vi "GetGamePiece.vi"() -> (0 "tx":dbl, 1 "ty":dbl, 2 "piece?":string, 3 "Vision Target Valid [t-?]":bool, 4 "confidence":dbl, 6 "Vision Timestamp (ms)":u32)   [LabVIEW 2020]
doc: "Reads the raw data from the LimeLight camera assigned to detecting AprilTags. Performs some minor transformations, conducts intial validity checks, and estimates the vision data timestamp."
uses:
  2d64956e-cf35-4d84-838e-e30eff74bf58.vi
  <vilib>/Rock Robotics/Network Tables/NT Read Number.vi
  GlobalDriverStationData.vi
  <vilib>/Rock Robotics/Network Tables/NT Read Numeric Array.vi
  <vilib>/Rock Robotics/Network Tables/NT Read String.vi
  GlobalPoseAndTargeting.vi
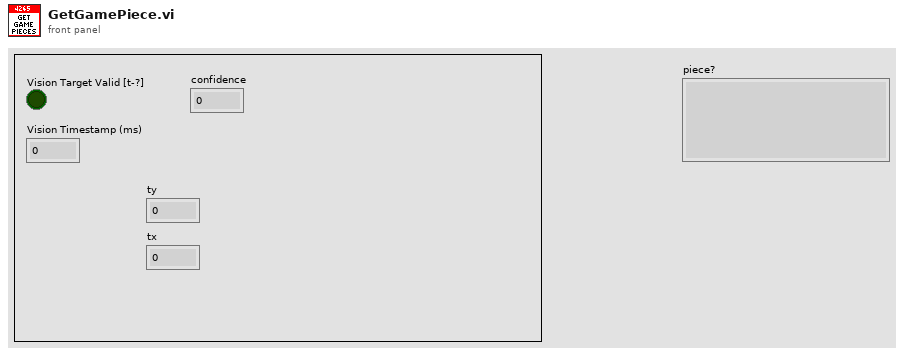
[diagram p1: front panel]
types:
  T1 = enum16{"Boot Up", "Camera Override", "AprilTags", "Gamepiece Tracking"}
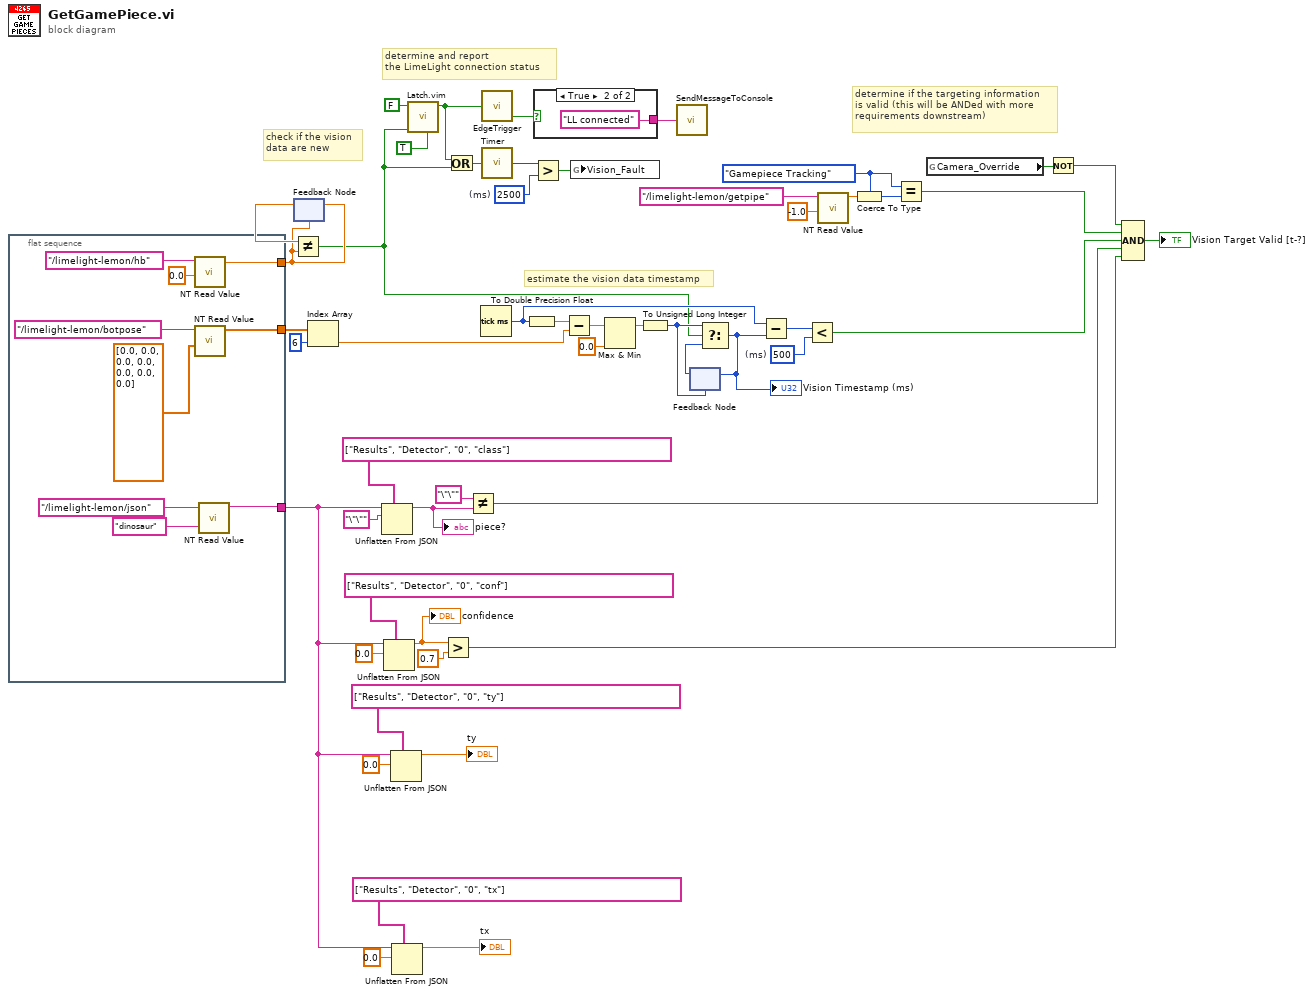
[diagram p0: block diagram]
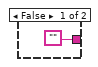
[diagram p2: hidden frame]
diagram:
  w24 = T1."Gamepiece Tracking"
  w35 = u32 2500  # (ms)
  w28 = u32 500  # (ms)
  # "determine and report\nthe LimeLight connection status"
  # "determine if the targeting information\nis valid (this will be ANDed with more\nrequirements downstream)"
  # "estimate the vision data timestamp"
  # "check if the vision\ndata are new"
  n1 = flat-sequence {
    tunnel: [w59] -> w26
    tunnel: [w56] -> w21
    tunnel: [w54] -> w1
    frame #0 {
      n2 = call-poly <vilib>:"NT Read Value.vi"("default value"=0.0 ("Default Value"), "name"="/limelight-lemon/hb" ("Name")) -> ("value"=w59:dbl)  [unwired: 7 in, 2 out]
      n3 = call-poly <vilib>:"NT Read Value.vi"("default value"=dbl[] [0.0, 0.0, 0.0, 0.0, 0.0, 0.0, 0.0], "name"="/limelight-lemon/botpose" ("Name")) -> ("value"=w56:dbl[])  [unwired: 7 in, 2 out]
      n4 = call-poly <vilib>:"NT Read Value.vi"("default value"="dinosaur", "name"="/limelight-lemon/json" ("Name")) -> ("value"=w54:string)  [unwired: 7 in, 2 out]
    }
  }
  n5 = feedback-in #1(w26) -> ()
  n6 = feedback #1(w26) -> (w37:dbl)
  n7 = Not Equal?(x=w37, y=w26) -> (x != y?=w25:bool)
  n8 = Index Array(array=w21, index=6) -> (element=w20:dbl)
  n9 = Unflatten From JSON(path=string[] ["Results", "Detector", "0", "class"], JSON string=w1, type and defaults="\"\"") -> (value=w2:string)  [unwired: 4 in, 1 out]
  "piece?" <- w2
  n10 = Unflatten From JSON(path=string[] ["Results", "Detector", "0", "conf"], JSON string=w1, type and defaults=0.0) -> (value=w10:dbl)  [unwired: 4 in, 1 out]
  "confidence" <- w10
  n11 = Unflatten From JSON(path=string[] ["Results", "Detector", "0", "ty"], JSON string=w1, type and defaults=0.0) -> (value=→"ty":dbl)  [unwired: 4 in, 1 out]
  n12 = Unflatten From JSON(path=string[] ["Results", "Detector", "0", "tx"], JSON string=w1, type and defaults=0.0) -> (value=→"tx":dbl)  [unwired: 4 in, 1 out]
  n13 = call "Latch.vim"("Default Value"=TRUE, "Latch Signal"=w25, "Latch Value"=FALSE) -> ("Latched"=w31:bool)  [unwired: 8 in]
  n14 = Greater?(x=w10, y=0.7 ("x")) -> (0:w12:bool)
  n15 = Or(x=w31, y=w25) -> (x .or. y?=w34:bool)
  n16 = Not Equal?(x="\"\"", y=w2) -> (x != y?=w3:bool)
  n17 = Tick Count (ms)() -> (millisecond timer value=w41:u32)
  n18 = call "EdgeTrigger.vi"("Input Signal"=w31) -> ("Falling Edge Trigger"=w29:bool)  [unwired: 2 out]
  n19 = call "Timer.vi"("Reset Timer"=w34) -> ("Time (ms)"=w36:u32)
  n20 = To Double Precision Float(number=w41) -> (double precision float=w46:dbl)
  n21 = Greater?(x=w36, y=w35) -> (0:w27:bool)
  n22 = case shown="True" w29 {
    tunnel: ["" "LL connected" ("Message")] -> w30
    frame False {
    }
    frame True {
    }
  }
  n23 = Subtract(x=w46, y=w20) -> (x-y=w45:dbl)
  n24 = global write "GlobalPoseAndTargeting.vi" "Vision_Fault"(w27) -> ()
  n25 = Max & Min(x=w45, y=0.0) -> (max(x,y)=w43:dbl)  [unwired: 1 out]
  n26 = To Unsigned Long Integer(number=w43) -> (unsigned 32bit integer=w42:u32)
  n27 = call "SendMessageToConsole.vi"("Message String"=w30) -> ()  [unwired: 1 in]
  n28 = feedback #2(w42) -> (w47:u32)
  n29 = Select(t=w42, s=w25, f=w47) -> (s? t:f=w18:u32)
  "Vision Timestamp (ms)" <- w18
  n30 = feedback-in #2(w18) -> ()
  n31 = Subtract(x=w41, y=w18) -> (x-y=w40:u32)
  n32 = Less?(x=w40, y=w28) -> (x < y?=w23:bool)
  n33 = call-poly <vilib>:"NT Read Value.vi"("default value"=-1.0 ("Default Value"), "name"="/limelight-lemon/getpipe" ("Name")) -> ("value"=w50:dbl)  [unwired: 7 in, 2 out]
  n34 = Coerce To Type(0:w50, 1:w24) -> (2:w49:T1)
  n35 = Equal?(x=w24, y=w49) -> (x = y?=w48:bool)
  n36 = global read "GlobalDriverStationData.vi" "Camera_Override"() -> (w39:bool)
  n37 = Not(x=w39) -> (.not. x?=w38:bool)
  n38 = Compound Arithmetic op=AND(w38, w48, w23, w3, w12) -> (→"Vision Target Valid [t-?]":bool)
